vi "字符检测CCD1-1.vi"(8 "error in (no error)":errorcluster caption="错误输入（无错误）", 11 "名称或相对路径":string="Template Program") -> (0 "error in (no error) 2":errorcluster caption="错误输入（无错误）")   [LabVIEW 2017]
uses:
  Picture/SaveButtom.ctl
  Global System.vi
  <vilib>/Utility/xml.llb/Write to XML File(string).vi
panel:
  in  "获取图像":bool
  in  "ROI获取":bool
  in  "创建模板":bool
  in  "保存图像":bool
  out "添加的路径":path
  in  "刷新":bool
  in  "测试按钮":bool
  in  "保存按钮":bool
  in  "Main":enum32{"主参数", "字符检测参数 ", "测试效果"}(tab)
  in  "字符检测基础参数":T1={"IsNorImage"=TRUE, "Exposure Values"=100289, "ImagePath"=path "C:/Users/hedongpo/Desktop/514-hdp/Alignment Assemble System/Test Picture/B/3.bmp"} caption="参数界面" {"Exposure Values" scale=0.0..200000.0}
  in  "Angle (degrees)":sgl=93.5
  in  "字符识别参数":T3={"Parameters (OCR/OCV 1)"={"Threshold Data"={"Method"=enum."Local", "Looking for"=1, "Color Mode"=0, "Kernel Size"={"Width"=32, "Height"=32}, "Ranges"=[{"Min"=1, "Max"=255}]}, "Reject Border"=TRUE, "Number \nOf Erosions"=0, "Size & Spacing"={"Segment Algorithm"=0, "Min Bounding Rect Width"=1, "Max Bounding Rect Width"=65536, "Min Bounding Rect Height"=1, "Max Bounding Rect Height"=65536, "Min Character Size"=20, "Max Character Size"=65536, "Min Char Spacing"=1, "Max Horiz Element Spacing"=1, "Max Vert Element Spacing"=0, "Max Space Distance"=65536}, "Read Options"={"Read Strategy"=1, "Read Resolution"=2, "Scale Dependant"=FALSE, "Aspect Ratio"=400, "Acceptance Level"=700, "Substitution Character"="?", "MultiLine"=TRUE}, "Valid Characters"=[], "Use Text Pattern"=FALSE, "Orientation"=0, "# Lines Expected"=0, "Number of Blocks"=4}, "File Path "=path "D:/Inspect System -2/Source Code/Template Program/字符模板.abc", "Rectangle"={"Left"=0, "Top"=0, "Right"=0, "Bottom"=0, "Rotation"=0.0}, "字符长度判定"=0.0} {"Rectangle"."Rotation" min=-90.0 max=90.0 step=1.0 format="%.2f"; "Rectangle"."Left" scale=0.0..1024.0; "Rectangle"."Right" scale=0.0..1024.0; "Parameters (OCR/OCV 1)"."Threshold Data"."Looking for" items=["Light on Dark", "Dark on Light"]; "Parameters (OCR/OCV 1)"."Threshold Data"."Color Mode" items=["RGB", "HSL", "HSV", "HSI"]; "Parameters (OCR/OCV 1)"."Size & Spacing"."Segment Algorithm" items=["None", "Shortest Segment", "Legacy Auto Split"]; "Parameters (OCR/OCV 1)"."Read Options"."Read Strategy" items=["Aggressive", "Conservative"]; "Parameters (OCR/OCV 1)"."Read Options"."Read Resolution" items=["Low", "Medium", "High"]; "Parameters (OCR/OCV 1)"."Valid Characters"."Pre-defined characters" items=["Any Character", "User-defined Characters", "Alphabetic", "Alphanumeric", "Uppercase Letters", "Lowercase Letters", "Decimal Digits", "Hexadecimal Digits", "Pattern", "Force Space"]; "Parameters (OCR/OCV 1)"."Orientation" items=["Baseline inside", "Baseline outside"]}
  out "原始图像":T4(plugin-control)
  out "String (OCR/OCV 1)":string
  out "路径输出":path
  in  "Vision Paramter Save Buttom":T5
  out "system time":string
  in  "取消按钮":bool
  # "85"
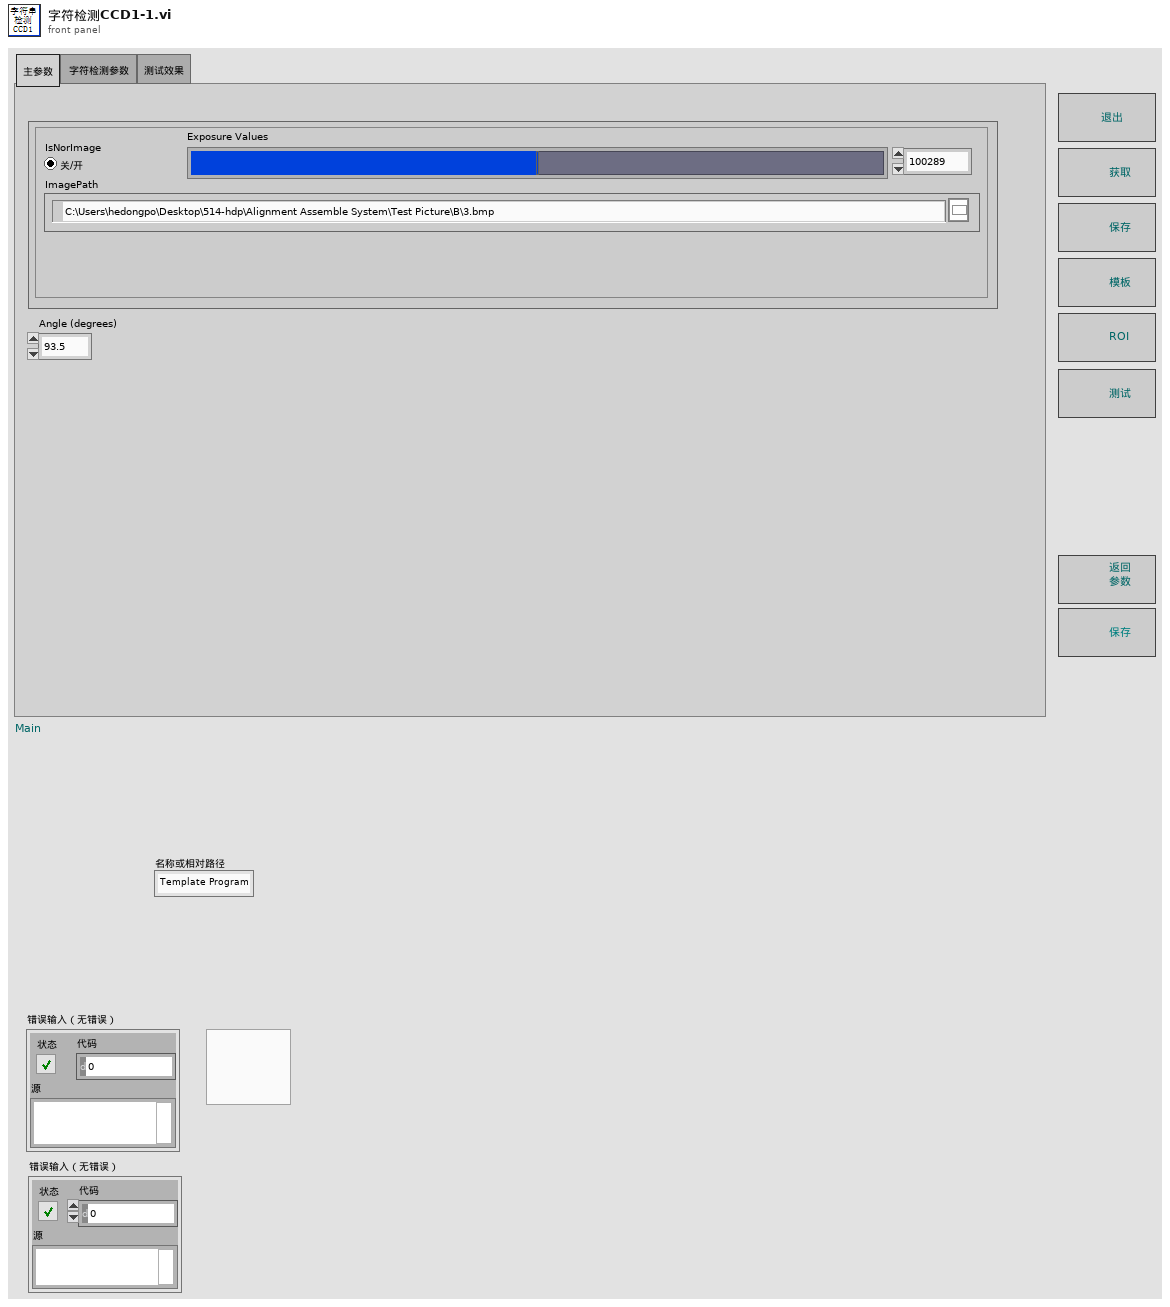
[diagram p1: front panel]
types:
  T1 = cluster{"IsNorImage":bool, "Exposure Values":u32, "ImagePath":path}
  T2 = typedef "IMAQ Rectangle" = cluster{"Left":i32, "Top":i32, "Right":i32, "Bottom":i32, "Rotation":dbl}
  T3 = cluster{"Parameters (OCR/OCV 1)":cluster{"Threshold Data":cluster{"Method":enum16{"Fixed Range", "Uniform", "Linear", "Non Linear", "Local", "Color"}, "Looking for":u32, "Color Mode":u32, "Kernel Size":cluster{"Width":i32, "Height":i32}, "Ranges":cluster{"Min":i32, "Max":i32}[]}, "Reject Border":bool, "Number \nOf Erosions":i32, "Size & Spacing":cluster{"Segment Algorithm":u16, "Min Bounding Rect Width":i32, "Max Bounding Rect Width":i32, "Min Bounding Rect Height":i32, "Max Bounding Rect Height":i32, "Min Character Size":i32, "Max Character Size":i32, "Min Char Spacing":i32, "Max Horiz Element Spacing":i32, "Max Vert Element Spacing":i32, "Max Space Distance":i32}, "Read Options":cluster{"Read Strategy":i32, "Read Resolution":i32, "Scale Dependant":bool, "Aspect Ratio":i32, "Acceptance Level":i32, "Substitution Character":string, "MultiLine":bool}, "Valid Characters":cluster{"Pre-defined characters":i32, "User-defined characters":string}[], "Use Text Pattern":bool, "Orientation":u32, "# Lines Expected":u32, "Number of Blocks":i32}, "File Path ":path, "Rectangle":T2, "字符长度判定":dbl}
  T4 = typedef "IMAQ Image.ctl" = refnum<image>
  T5 = typedef "SaveButtom.ctl" = bool
  T6 = cluster{"index":i32, "this vi":refnum<vi>, "error out":errorcluster}
  T7 = cluster{"master data":string, "priority":u16, "secondary data":string[]}
  T8 = cluster{"case name":string[], "queue array":refnum<queue>[]}
  T9 = cluster{"Global Rectangle":i32[], "Contours":cluster{"Contour Type":u32, "ROI Type":u32, "Points":i32[]}[]}
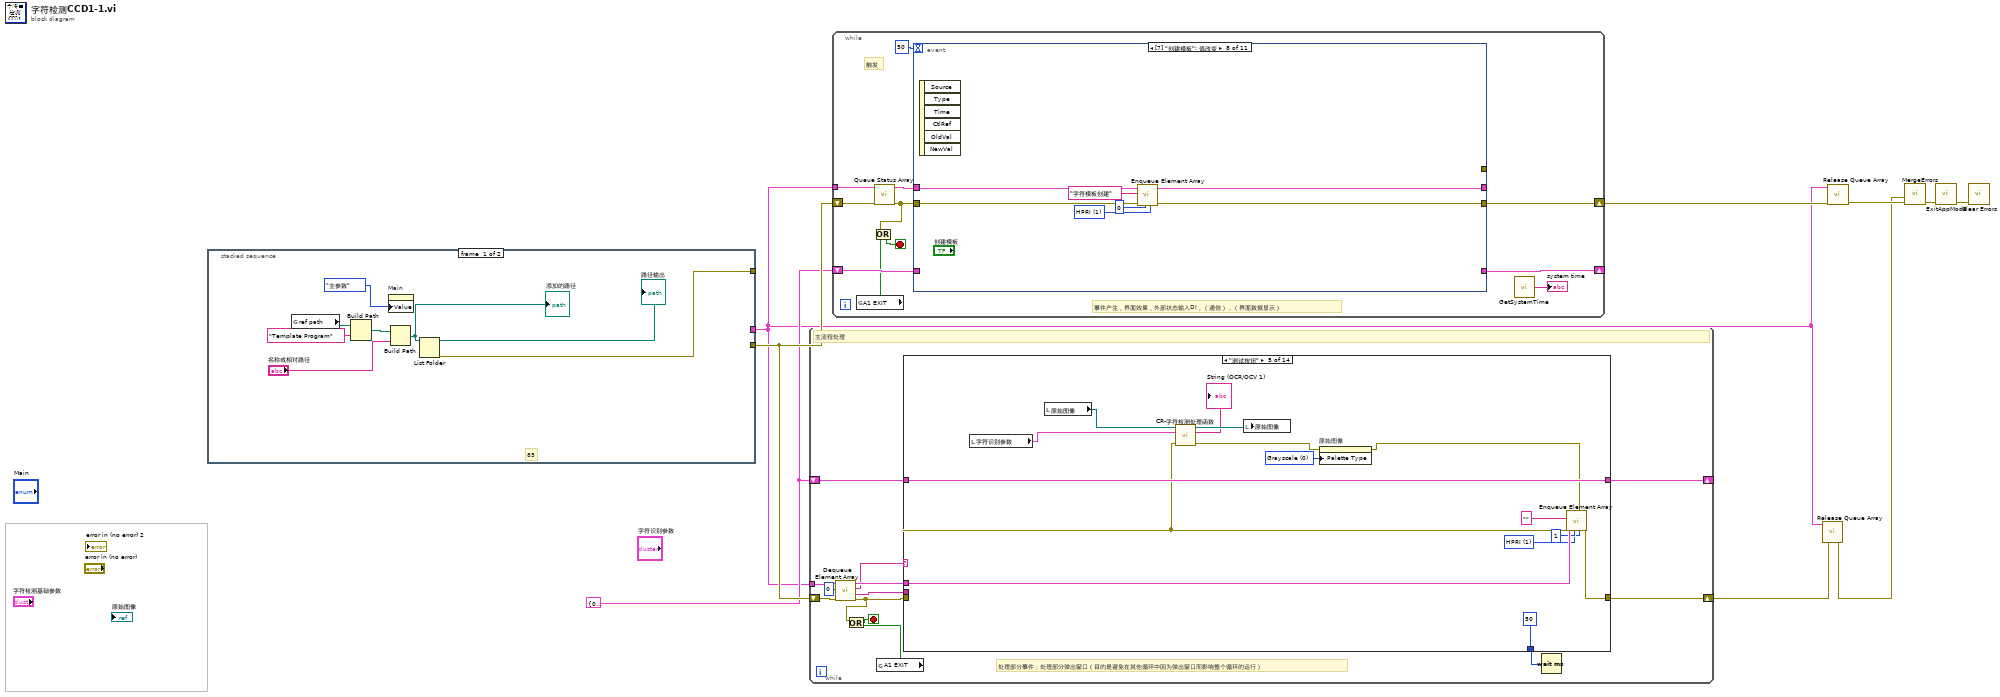
[diagram p0: block diagram]
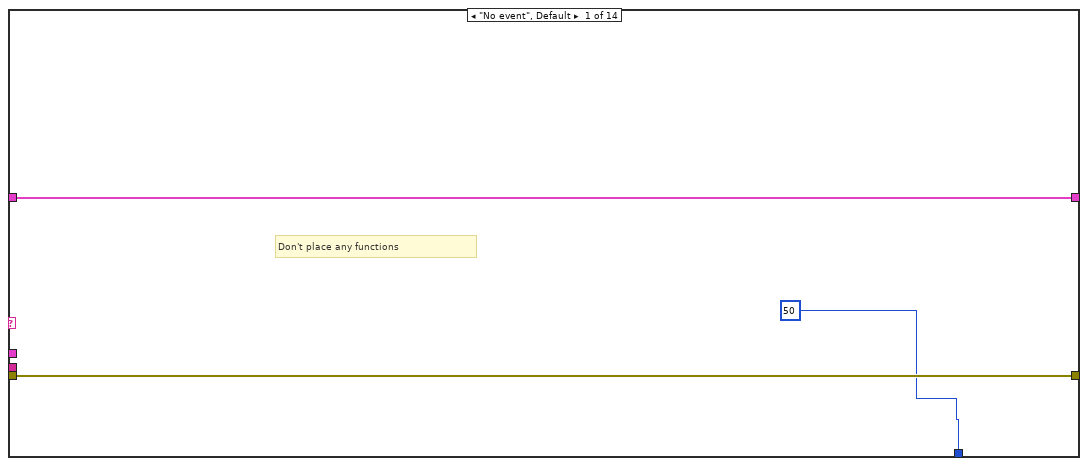
[diagram p2: hidden frame]
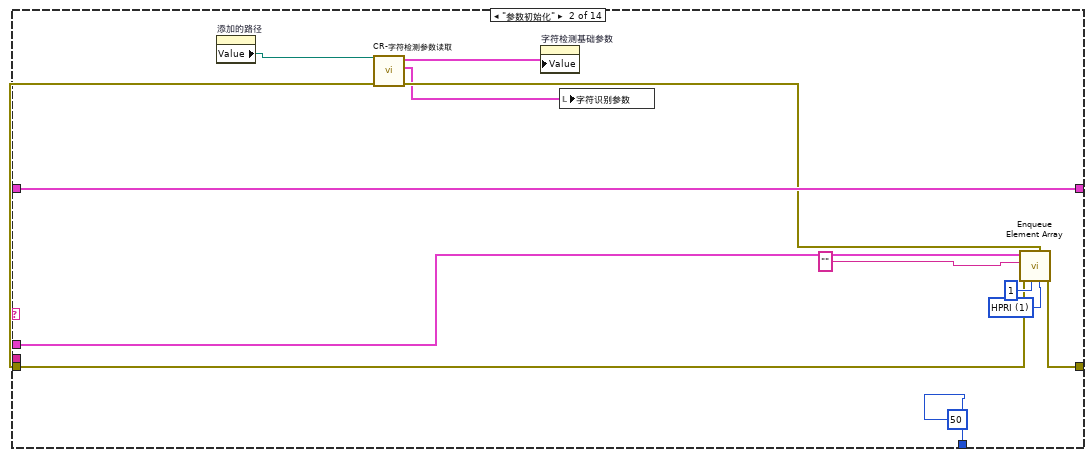
[diagram p3: hidden frame]
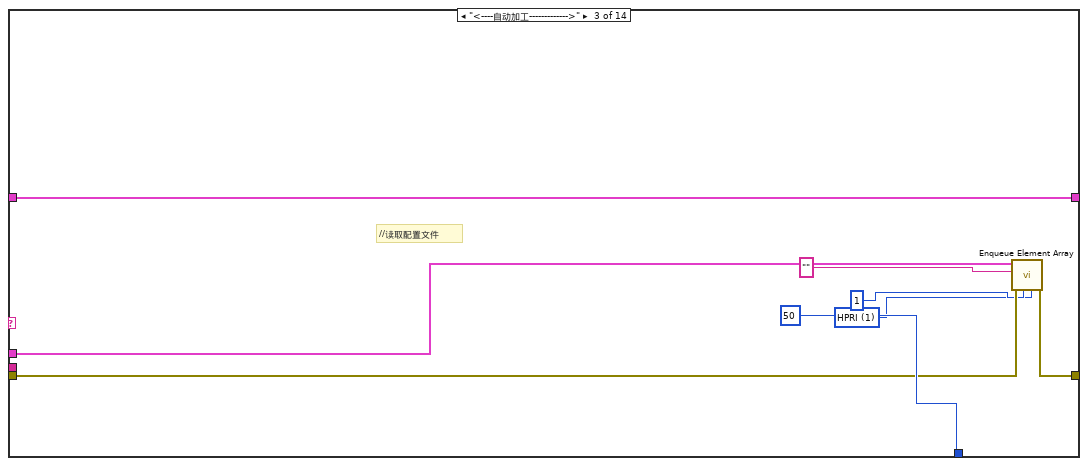
[diagram p4: hidden frame]
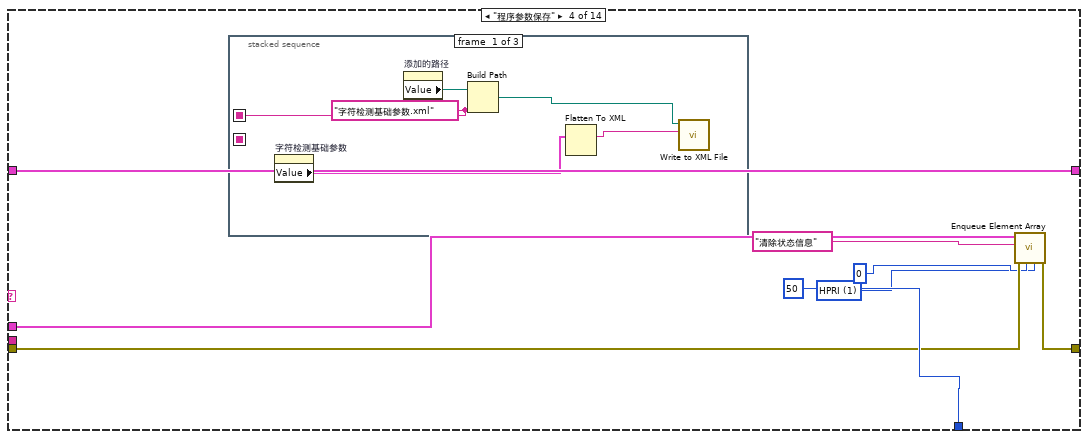
[diagram p5: hidden frame]
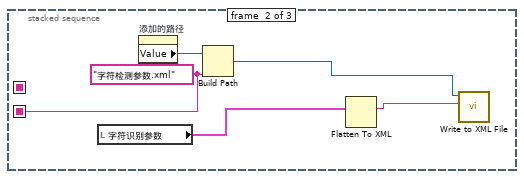
[diagram p6: hidden frame]
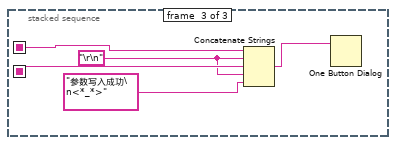
[diagram p7: hidden frame]
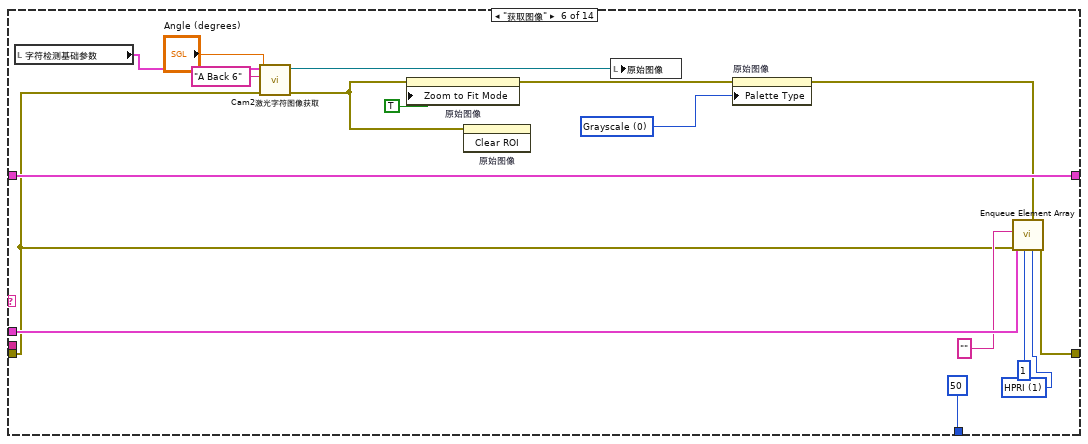
[diagram p8: hidden frame]
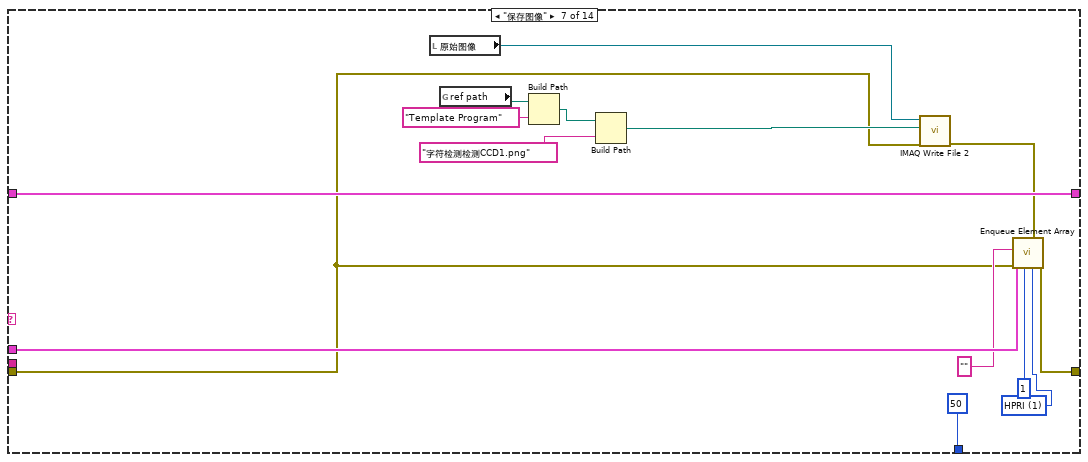
[diagram p9: hidden frame]
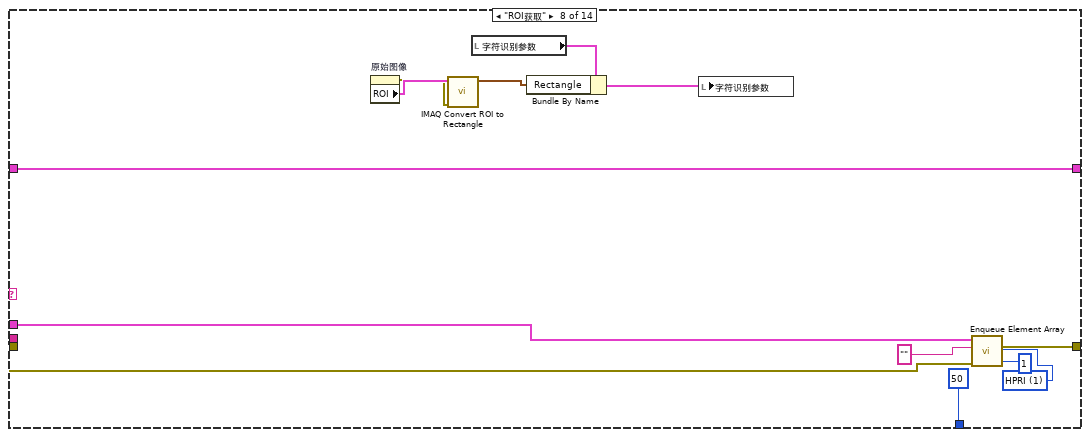
[diagram p10: hidden frame]
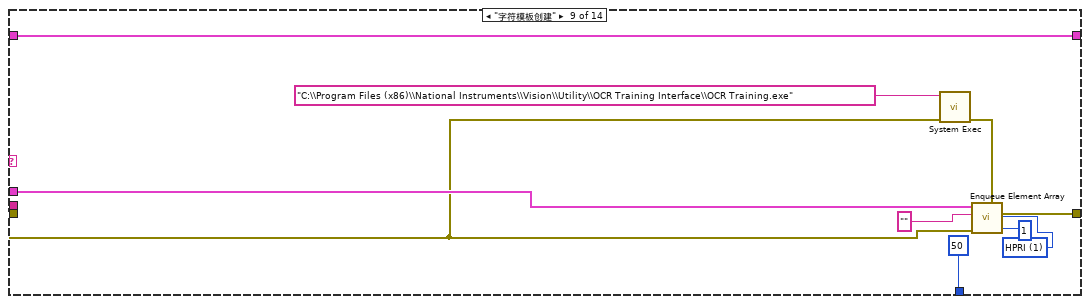
[diagram p11: hidden frame]
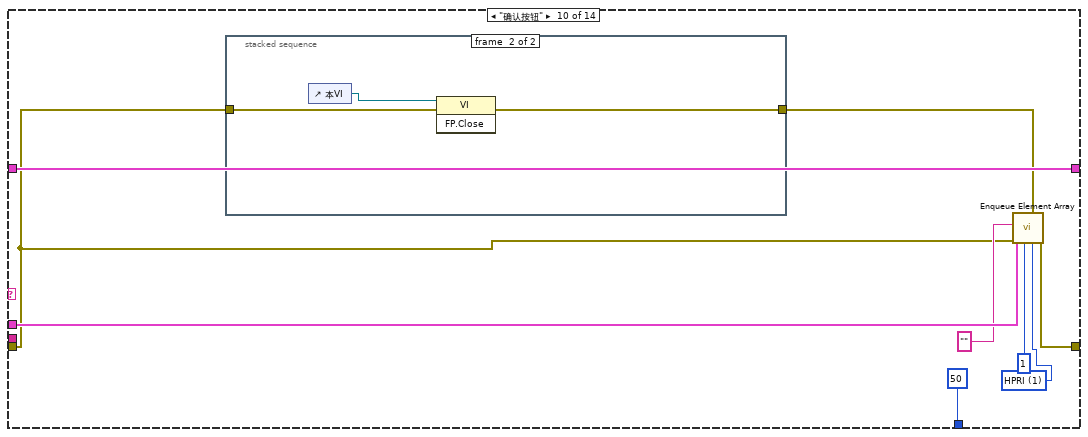
[diagram p12: hidden frame]
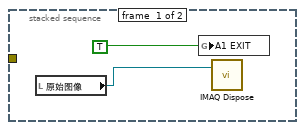
[diagram p13: hidden frame]
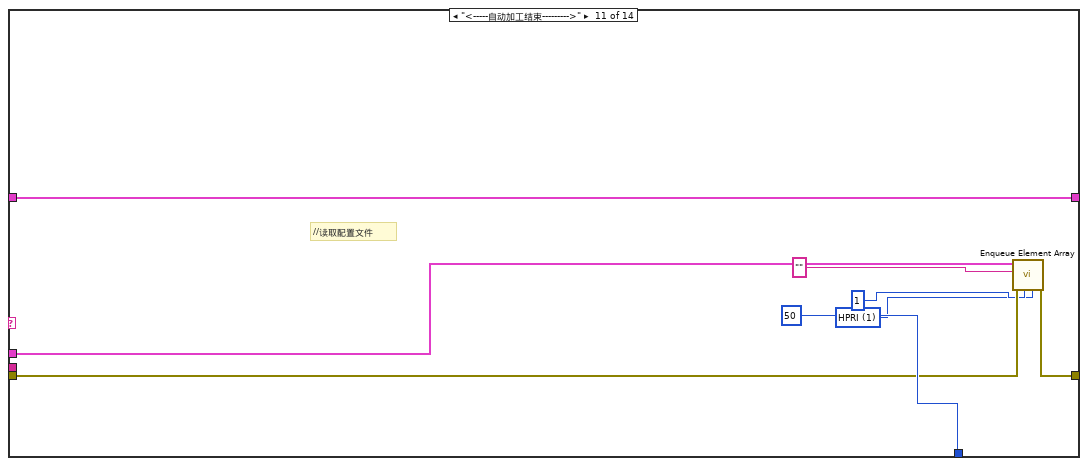
[diagram p14: hidden frame]
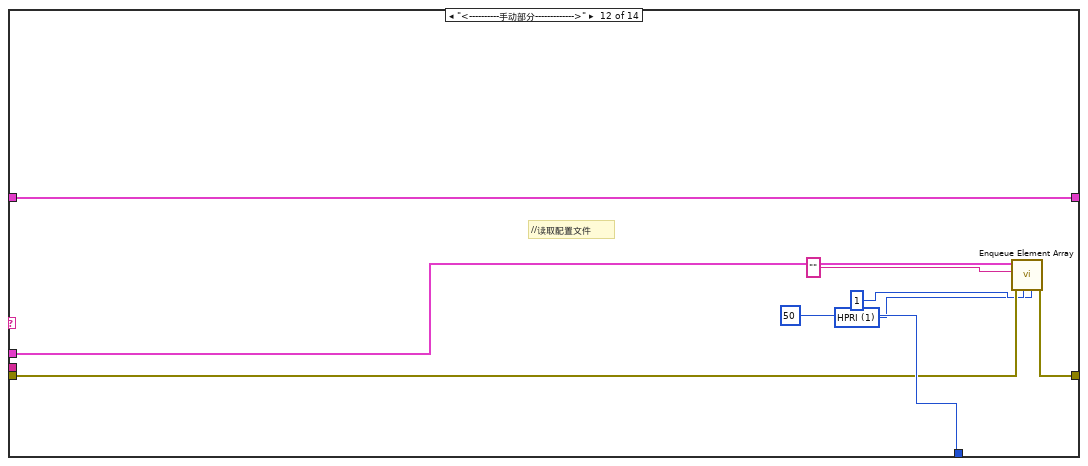
[diagram p15: hidden frame]
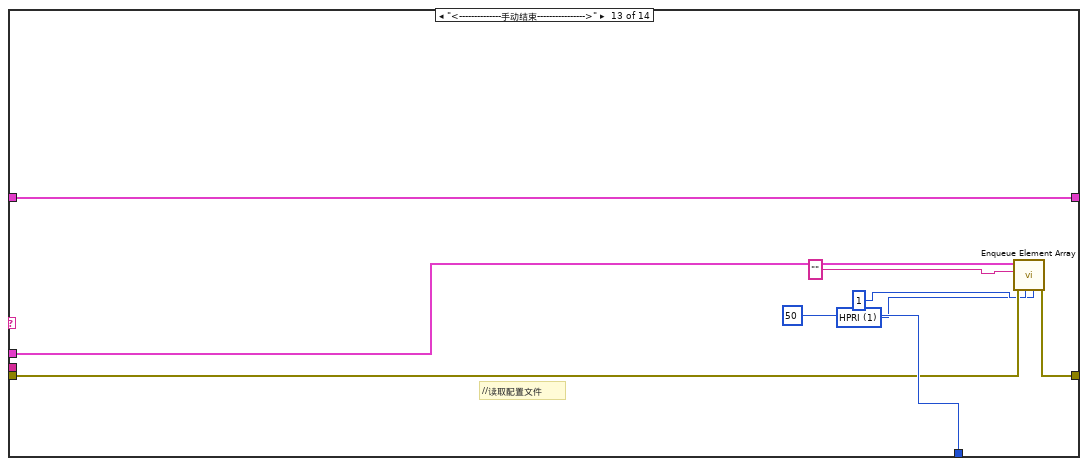
[diagram p16: hidden frame]
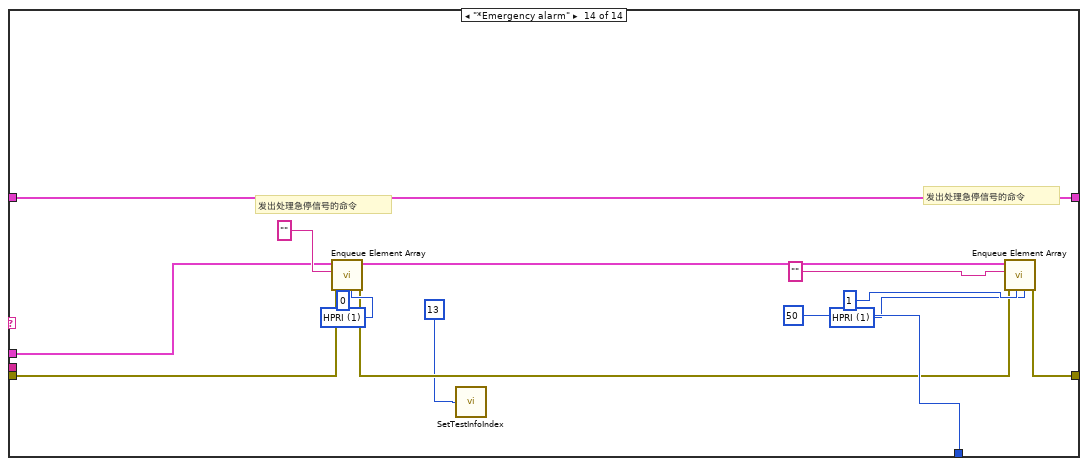
[diagram p17: hidden frame]
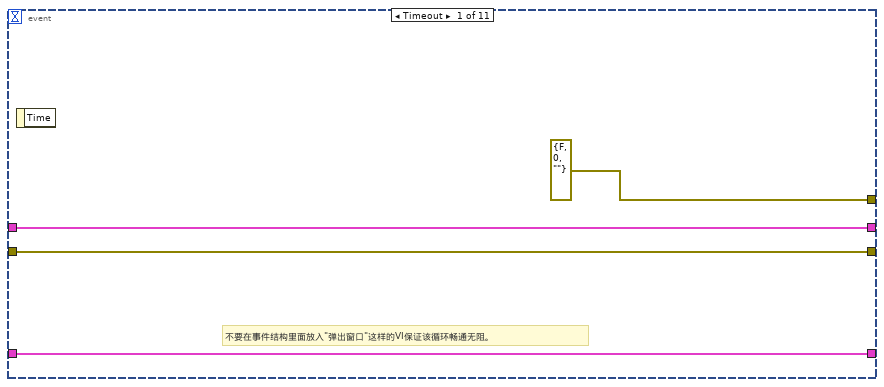
[diagram p18: hidden frame]
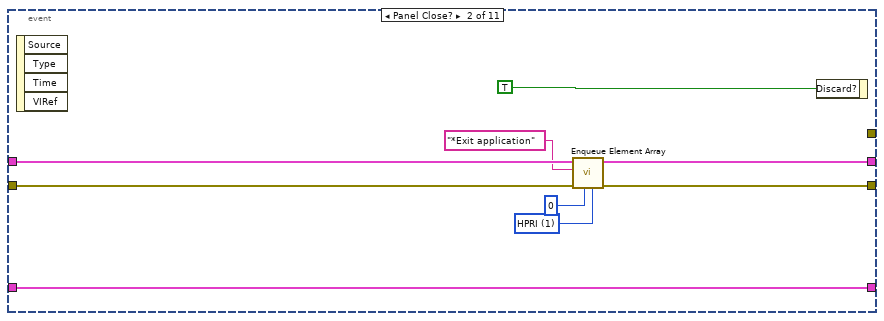
[diagram p19: hidden frame]
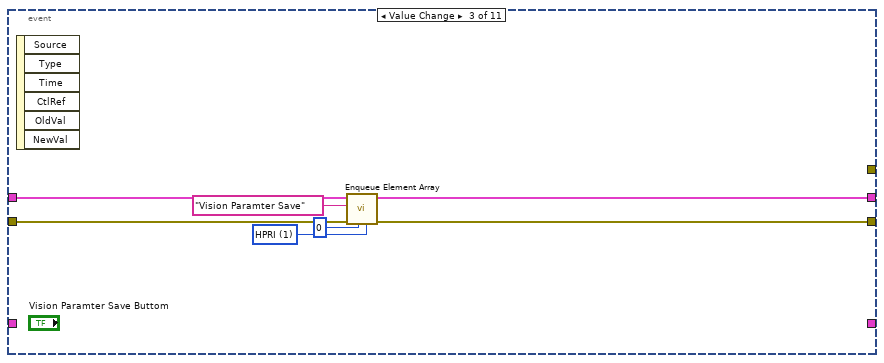
[diagram p20: hidden frame]
diagram:
  w4 = T6 {"index"=0, "this vi"=refnum, "error out"={"status"=FALSE, "code"=0, "source"=""}} ("parameter buffer")
  # "85"
  n1 = stacked-sequence {
    tunnel: [w15 _] -> _
    tunnel: [_ w19] -> w5
    tunnel: [_ w18] -> w1
    frame #0 {
      n2 = global read "Global System.vi" "ref path"() -> (w13:path)
      n3 = Build Path(base path=w13, name or relative path="Template Program" ("名称或相对路径")) -> (appended path=w11:path)
      n4 = property on="Main" class="TabCtl (严格)"("Value"=enum32{"主参数", "字符检测参数 ", "测试效果"}."主参数" ("Main")) -> ()  [unwired: 2 in, 2 out]
      n5 = Build Path(base path=w11, name or relative path="名称或相对路径") -> (appended path=w17:path)
      "添加的路径" <- w17
      n6 = List Folder(path=w17) -> (path out=→"路径输出":path, error out=w15:errorcluster)  [unwired: 3 in, 2 out]
    }
    frame #1 {
      w27 = string[] ["comm queue1", "data queue 11", "data queue 12", "data queue 13", "data queue 14"]  # queue name
      w28 = 4  # queue num
      w29 = T7 {"master data"="", "priority"=0, "secondary data"=[]}  # element data type
      n7 = call "Obtain Queue Array.vi"("queue name"=w27, "element data type"=w29, "queue num"=w28) -> ("error out"=w23:errorcluster, "queue out"=w24:T8)  [unwired: 2 in, 1 out]
      n8 = call "Enqueue Element Array.vi"("queue index"=0, "error in"=w23, "master data"="参数初始化", "queue in"=w24) -> ("error out"=w22:errorcluster, "queue out"=w21:T8)  [unwired: 6 in]
      n9 = disable-structure shown="启用" {
        disable-tunnel: w22 -> [w35 w36]
        disable-tunnel: w21 -> [w34 w37]
        disable-tunnel: "Loading Variable" ("master data") -> [w33 _]
        disable-tunnel: [w31 w36] -> w19
        disable-tunnel: [w30 w37] -> w18
        frame Disabled {
          n10 = call "Enqueue Element Array.vi"("queue index"=12, "error in"=w35, "master data"=w33, "queue in"=w34) -> ("error out"=w31:errorcluster, "queue out"=w30:T8)  [unwired: 6 in]
        }
        frame Enabled {
        }
      }
    }
  }
  n11 = while {
    shift-right: [w50] -> w3
    shift-left: w5 -> [w41]
    shift-right: [w47] -> _
    shift-left: w4 -> [w48]
    tunnel: w1 -> [w43]
    stop <- w38 stop-if-true
    # "处理部分事件；处理部分弹出窗口（目的是避免在其他循环中因为弹出窗口而影响整个循环的运行）"
    # "主流程处理"
    n12 = call "Dequeue Element Array.vi"("queue in"=w43, "queue index"=0, "error in"=w41) -> ("queue out"=w46:T8, "master data"=w45:string, "secondary data"=w44:string[], "error out"=w40:errorcluster)  [unwired: 2 in, 1 out]
    n13 = global read "Global System.vi" "A1 EXIT"() -> (w39:bool)
    n14 = Or(x=w40, y=w39) -> (x .or. y?=w38:bool)
    n15 = case shown="\"测试按钮\"" w45 {
      tunnel: w46 -> [_ w64 w72 w74 w110 w127 w142 w155 w165 w174 w187 w195 w203 w209]
      tunnel: w40 -> [w52 w58 w68 w78 w104 w118 w130 w149 w159 w168 w183 w191 w199 w206]
      tunnel: [w52 w63 w71 w80 w109 w126 w141 w154 w164 w173 w186 w194 w202 w217] -> w50
      tunnel: [50 50 50 50 50 50 50 50 50 50 50 50 50 50] -> w49
      tunnel: w48 -> [w53 w59 w69 w75 w105 w122 w137 w150 w160 w169 w184 w192 w200 w215]
      tunnel: [w53 w59 w69 w75 w105 w122 w137 w150 w160 w169 w184 w192 w200 w215] -> w47
      tunnel: w44 -> [_ _ _ _ _ _ _ _ _ _ _ _ _ _]
      frame "No event", Default {
        # "Don't place any functions"
      }
      frame "参数初始化" {
        w60 = u16 1 items=["HPRI"=1, "LPRI"=0] ("priority")
        n16 = property on="添加的路径" class="Path"() -> ("Value"=w56:path)  [unwired: 2 in, 2 out]
        n17 = call "CR-字符检测参数读取.vi"("error in (no error)"=w58, "基路径"=w56) -> ("error out"=w57:errorcluster, "字符识别参数"=w54:T3, "字符检测基础参数"=w55:T1)  [unwired: 6 in]
        n18 = property on="字符检测基础参数" class="Clust (严格)"("Value"=w55) -> ()  [unwired: 2 in, 2 out]
        n19 = local write "字符识别参数"(w54) -> ()
        n20 = call "Enqueue Element Array.vi"("priority"=w60, "device error in"=w57, "queue index"=1, "error in"=w58, "master data"="" ("Element 1"), "queue in"=w64) -> ("error out"=w63:errorcluster)  [unwired: 4 in, 1 out]
      }
      frame "<----自动加工------------->" {
        w66 = u16 1 items=["HPRI"=1, "LPRI"=0] ("priority")
        # "//读取配置文件"
        n21 = call "Enqueue Element Array.vi"("priority"=w66, "queue index"=1, "error in"=w68, "master data"="" ("Element 1"), "queue in"=w72) -> ("error out"=w71:errorcluster)  [unwired: 5 in, 1 out]
      }
      frame "程序参数保存" {
        w76 = u16 1 items=["HPRI"=1, "LPRI"=0] ("priority")
        n22 = stacked-sequence {
          seq-local: [w82 _ _] -> [_ _ w95]
          seq-local: [_ w91 _] -> [_ _ w93]
          frame #0 {
            w82 = "字符检测基础参数.xml" ("名称或相对路径")
            n23 = property on="字符检测基础参数" class="Clust (严格)"() -> ("Value"=w85:T1)  [unwired: 2 in, 2 out]
            n24 = property on="添加的路径" class="Path"() -> ("Value"=w86:path)  [unwired: 2 in, 2 out]
            n25 = Build Path(base path=w86, name or relative path=w82) -> (appended path=w83:path)
            n26 = Flatten To XML(anything=w85) -> (xml string=w84:string)
            n27 = call-poly <vilib>:"Write to XML File.vi"("XML Input"=w84, "XML File Path"=w83) -> ()  [unwired: 7 in, 3 out]
          }
          frame #1 {
            w91 = "字符检测参数.xml" ("名称或相对路径")
            n28 = local read "字符识别参数"() -> (w87:T3)
            n29 = property on="添加的路径" class="Path"() -> ("Value"=w90:path)  [unwired: 2 in, 2 out]
            n30 = Build Path(base path=w90, name or relative path=w91) -> (appended path=w88:path)
            n31 = Flatten To XML(anything=w87) -> (xml string=w89:string)
            n32 = call-poly <vilib>:"Write to XML File.vi"("XML Input"=w89, "XML File Path"=w88) -> ()  [unwired: 7 in, 3 out]
          }
          frame #2 {
            w92 = "\r\n"
            n33 = Concatenate Strings(w95, w92, w93, w92, "参数写入成功\n<*_*>" ("消息")) -> (w94:string)
            n34 = One Button Dialog(message=w94) -> ()  [unwired: 1 in, 1 out]
          }
        }
        n35 = call "Enqueue Element Array.vi"("priority"=w76, "queue index"=0, "error in"=w78, "master data"="清除状态信息" ("Element 1"), "queue in"=w74) -> ("error out"=w80:errorcluster)  [unwired: 5 in, 1 out]
      }
      frame "测试按钮" {
        w100 = u32 0 items=["Grayscale", "Binary", "Gradient", "Rainbow", "Temperature", "User Defined", "Binary 16 Bit", "Gradient 16 Bit", "Rainbow 16 Bit", "Temperature 16 Bit", "User Defined 16 Bit"] ("Palette:Palette Type")
        w106 = u16 1 items=["HPRI"=1, "LPRI"=0] ("priority")
        n36 = local read "字符识别参数"() -> (w97:T3)
        n37 = local read "原始图像"() -> (w101:T4)
        n38 = call "CR-字符检测处理函数.vi"("error in (no error)"=w104, "字符识别参数"=w97, "Image in"=w101) -> ("error out"=w99:errorcluster, "String (OCR/OCV 1)"=→"String (OCR/OCV 1)":string, "Image out"=w103:T4)  [unwired: 4 in, 2 out]
        n39 = local write "原始图像"(w103) -> ()
        n40 = property on="原始图像" class="ImageControl"(error in=w99, "Palette Type"=w100) -> (error out=w98:errorcluster)  [unwired: 1 in, 1 out]
        n41 = call "Enqueue Element Array.vi"("priority"=w106, "device error in"=w98, "queue index"=1, "error in"=w104, "master data"="" ("Element 1"), "queue in"=w110) -> ("error out"=w109:errorcluster)  [unwired: 4 in, 1 out]
      }
      frame "获取图像" {
        w115 = u32 0 items=["Grayscale", "Binary", "Gradient", "Rainbow", "Temperature", "User Defined", "Binary 16 Bit", "Gradient 16 Bit", "Rainbow 16 Bit", "Temperature 16 Bit", "User Defined 16 Bit"] ("Palette:Palette Type")
        w123 = u16 1 items=["HPRI"=1, "LPRI"=0] ("priority")
        n42 = local read "字符检测基础参数"() -> (w120:T1)
        n43 = call "Cam2激光字符图像获取.vi"("error in (no error)"=w118, "Angle (degrees)"="Angle (degrees)", "Image Name"="A Back 6", "ParamsUI"=w120) -> ("error out"=w116:errorcluster, "Image out"=w119:T4)  [unwired: 3 in, 3 out]
        n44 = property on="原始图像" class="ImageControl"(error in=w116, "Zoom to Fit Mode"=TRUE) -> (error out=w114:errorcluster)  [unwired: 1 in, 1 out]
        n45 = invoke on="原始图像" class="ImageControl" method="Clear ROI"(error in=w116) -> ()  [unwired: 2 in, 3 out]
        n46 = local write "原始图像"(w119) -> ()
        n47 = property on="原始图像" class="ImageControl"(error in=w114, "Palette Type"=w115) -> (error out=w113:errorcluster)  [unwired: 1 in, 1 out]
        n48 = call "Enqueue Element Array.vi"("priority"=w123, "device error in"=w113, "queue index"=1, "error in"=w118, "master data"="" ("Element 1"), "queue in"=w127) -> ("error out"=w126:errorcluster)  [unwired: 4 in, 1 out]
      }
      frame "保存图像" {
        w138 = u16 1 items=["HPRI"=1, "LPRI"=0] ("priority")
        n49 = local read "原始图像"() -> (w129:T4)
        n50 = global read "Global System.vi" "ref path"() -> (w136:path)
        n51 = Build Path(base path=w136, name or relative path="Template Program" ("名称或相对路径")) -> (appended path=w134:path)
        n52 = Build Path(base path=w134, name or relative path="字符检测检测CCD1.png" ("名称或相对路径")) -> (appended path=w132:path)
        n53 = call-poly "IMAQ Write File 2"("error in (no error)"=w130, "File Path"=w132, "Image"=w129) -> ("error out"=w131:errorcluster)  [unwired: 7 in, 1 out]
        n54 = call "Enqueue Element Array.vi"("priority"=w138, "device error in"=w131, "queue index"=1, "error in"=w130, "master data"="" ("Element 1"), "queue in"=w142) -> ("error out"=w141:errorcluster)  [unwired: 4 in, 1 out]
      }
      frame "ROI获取" {
        w151 = u16 1 items=["HPRI"=1, "LPRI"=0] ("priority")
        n55 = property on="原始图像" class="ImageControl"() -> (error out=w145:errorcluster, "ROI"=w146:T9)  [unwired: 2 in, 1 out]
        n56 = call "IMAQ Convert ROI to Rectangle"("error in (no error)"=w145, "ROI Descriptor"=w146) -> ("Rectangle"=w144:T2)  [unwired: 7 in, 1 out]
        n57 = local read "字符识别参数"() -> (w148:T3)
        n58 = Bundle By Name(cluster=w148, "Rectangle"=w144) -> (w147:T3)
        n59 = local write "字符识别参数"(w147) -> ()
        n60 = call "Enqueue Element Array.vi"("priority"=w151, "queue index"=1, "error in"=w149, "master data"="" ("Element 1"), "queue in"=w155) -> ("error out"=w154:errorcluster)  [unwired: 5 in, 1 out]
      }
      frame "字符模板创建" {
        w161 = u16 1 items=["HPRI"=1, "LPRI"=0] ("priority")
        n61 = call <vilib>:"System Exec.vi"("error in (no error)"=w159, "command line"="C:\\Program Files (x86)\\National Instruments\\Vision\\Utility\\OCR Training Interface\\OCR Training.exe") -> ("error out"=w158:errorcluster)  [unwired: 6 in, 3 out]
        n62 = call "Enqueue Element Array.vi"("priority"=w161, "device error in"=w158, "queue index"=1, "error in"=w159, "master data"="" ("Element 1"), "queue in"=w165) -> ("error out"=w164:errorcluster)  [unwired: 4 in, 1 out]
      }
      frame "确认按钮" {
        w170 = u16 1 items=["HPRI"=1, "LPRI"=0] ("priority")
        n63 = stacked-sequence {
          tunnel: w168 -> [_ w179]
          tunnel: [_ w178] -> w167
          frame #0 {
            n64 = local read "原始图像"() -> (w176:T4)
            n65 = global write "Global System.vi" "A1 EXIT"(TRUE ("EXIT")) -> ()
            n66 = call "IMAQ Dispose"("Image"=w176) -> ()  [unwired: 5 in, 1 out]
          }
          frame #1 {
            n67 = control-ref of="本VI"() -> (w180:refnum<vi>)
            n68 = invoke class="VI" method="FP.Close"(reference=w180, error in=w179) -> (error out=w178:errorcluster)  [unwired: 1 in, 2 out]
          }
        }
        n69 = call "Enqueue Element Array.vi"("priority"=w170, "device error in"=w167, "queue index"=1, "error in"=w168, "master data"="" ("Element 1"), "queue in"=w174) -> ("error out"=w173:errorcluster)  [unwired: 4 in, 1 out]
      }
      frame "<-----自动加工结束--------->" {
        w181 = u16 1 items=["HPRI"=1, "LPRI"=0] ("priority")
        # "//读取配置文件"
        n70 = call "Enqueue Element Array.vi"("priority"=w181, "queue index"=1, "error in"=w183, "master data"="" ("Element 1"), "queue in"=w187) -> ("error out"=w186:errorcluster)  [unwired: 5 in, 1 out]
      }
      frame "<----------手动部分------------->" {
        w189 = u16 1 items=["HPRI"=1, "LPRI"=0] ("priority")
        # "//读取配置文件"
        n71 = call "Enqueue Element Array.vi"("priority"=w189, "queue index"=1, "error in"=w191, "master data"="" ("Element 1"), "queue in"=w195) -> ("error out"=w194:errorcluster)  [unwired: 5 in, 1 out]
      }
      frame "<--------------手动结束---------------->" {
        w197 = u16 1 items=["HPRI"=1, "LPRI"=0] ("priority")
        # "//读取配置文件"
        n72 = call "Enqueue Element Array.vi"("priority"=w197, "queue index"=1, "error in"=w199, "master data"="" ("Element 1"), "queue in"=w203) -> ("error out"=w202:errorcluster)  [unwired: 5 in, 1 out]
      }
      frame "*Emergency alarm" {
        w212 = u16 1 items=["HPRI"=1, "LPRI"=0] ("priority")
        w213 = u16 1 items=["HPRI"=1, "LPRI"=0] ("priority")
        # "发出处理急停信号的命令"
        # "发出处理急停信号的命令"
        n73 = call "Enqueue Element Array.vi"("priority"=w212, "queue index"=0, "error in"=w206, "master data"="" ("Element 1"), "queue in"=w209) -> ("error out"=w207:errorcluster, "queue out"=w208:T8)  [unwired: 5 in]
        n74 = call "SetTestInfoIndex.vi"("test info index"=13) -> ()
        n75 = call "Enqueue Element Array.vi"("priority"=w213, "queue index"=1, "error in"=w207, "master data"="" ("Element 1"), "queue in"=w208) -> ("error out"=w217:errorcluster)  [unwired: 5 in, 1 out]
      }
    }
    n76 = Wait (ms)(milliseconds to wait=w49) -> ()  [unwired: 1 out]
  }
  n77 = while {
    shift-right: [w222] -> w6
    shift-left: w5 -> [w226]
    shift-right: [w224] -> _
    shift-left: w4 -> [w225]
    tunnel: w1 -> [w228]
    stop <- w219 stop-if-true
    # "触发"
    # "事件产生，界面效果，外部状态输入DI，（通信），（界面数据显示）"
    n78 = global read "Global System.vi" "A1 EXIT"() -> (w220:bool)
    n79 = call "Queue Status Array.vi"("error in (no error)"=w226, "queue in"=w228) -> ("error out"=w221:errorcluster, "queue out"=w223:T8)  [unwired: 4 in]
    n80 = Or(x=w221, y=w220) -> (x .or. y?=w219:bool)
    n81 = event shown="[7] \"创建模板\": 值改变" {
      selector: _ -> [_ _ _ _ _ _ _ _ _ _ _]
      dyn-events: _ -> [_ _ _ _ _ _ _ _ _ _ _]
      timeout: 50 -> [_ _ _ _ _ _ _ _ _ _ _]
      tunnel: w225 -> [w233 w241 _ _ _ _ _ _ _ _ _]
      tunnel: [w233 w241 _ _ _ _ _ _ _ _ _] -> w224
      tunnel: [errorcluster {"status"=FALSE, "code"=0, "source"=""} ("error out") _ _ _ _ _ _ _ _ _ _] -> _
      tunnel: w223 -> [w231 w240 w246 w253 w260 w268 w275 w282 w290 w298 w306]
      tunnel: w221 -> [w230 w239 w245 w252 w259 w267 w274 w281 w289 w297 w305]
      tunnel: [w230 w238 w243 w250 w257 w265 w272 w279 w287 w295 w303] -> w222
      tunnel: [w231 w237 w244 w251 w258 w266 w273 w280 w288 w296 w304] -> _
      event Timeout {
        # "不要在事件结构里面放入\"弹出窗口\"这样的VI保证该循环畅通无阻。"
        n82 = event-data() -> ()  [unwired: 1 in, 1 out]
      }
      event Panel Close? {
        w235 = u16 1 items=["HPRI"=1, "LPRI"=0] ("priority")
        n83 = event-data() -> ()  [unwired: 1 in, 4 out]
        n84 = call "Enqueue Element Array.vi"("priority"=w235, "queue index"=0, "error in"=w239, "master data"="*Exit application", "queue in"=w240) -> ("error out"=w238:errorcluster, "queue out"=w237:T8)  [unwired: 5 in]
        n85 = event-data("Discard?"=TRUE) -> ()  [unwired: 1 in, 1 out]
      }
      event Value Change {
        w248 = u16 1 items=["HPRI"=1, "LPRI"=0] ("priority")
        n86 = event-data() -> ()  [unwired: 1 in, 6 out]
        n87 = call "Enqueue Element Array.vi"("priority"=w248, "queue index"=0, "error in"=w245, "master data"="Vision Paramter Save", "queue in"=w246) -> ("error out"=w243:errorcluster, "queue out"=w244:T8)  [unwired: 5 in]
      }
      event "取消按钮": Value Change {
        w255 = u16 1 items=["HPRI"=1, "LPRI"=0] ("priority")
        n88 = event-data() -> ()  [unwired: 1 in, 6 out]
        n89 = call "Enqueue Element Array.vi"("priority"=w255, "queue index"=0, "error in"=w252, "master data"="确认按钮", "queue in"=w253) -> ("error out"=w250:errorcluster, "queue out"=w251:T8)  [unwired: 5 in]
      }
      event "保存按钮": Value Change {
        w262 = u16 1 items=["HPRI"=1, "LPRI"=0] ("priority")
        n90 = event-data() -> ()  [unwired: 1 in, 6 out]
        n91 = call "Enqueue Element Array.vi"("priority"=w262, "queue index"=0, "error in"=w259, "master data"="程序参数保存", "queue in"=w260) -> ("error out"=w257:errorcluster, "queue out"=w258:T8)  [unwired: 5 in]
      }
      event "获取图像": Value Change {
        w270 = u16 1 items=["HPRI"=1, "LPRI"=0] ("priority")
        n92 = event-data() -> ()  [unwired: 1 in, 6 out]
        n93 = property on="Main" class="TabCtl (严格)"("Value"=enum32{"主参数", "字符检测参数 ", "测试效果"}."测试效果" ("Main")) -> ()  [unwired: 2 in, 2 out]
        n94 = call "Enqueue Element Array.vi"("priority"=w270, "queue index"=0, "error in"=w267, "master data"="获取图像", "queue in"=w268) -> ("error out"=w265:errorcluster, "queue out"=w266:T8)  [unwired: 5 in]
      }
      event "保存图像": Value Change {
        w277 = u16 1 items=["HPRI"=1, "LPRI"=0] ("priority")
        n95 = event-data() -> ()  [unwired: 1 in, 6 out]
        n96 = call "Enqueue Element Array.vi"("priority"=w277, "queue index"=0, "error in"=w274, "master data"="保存图像", "queue in"=w275) -> ("error out"=w272:errorcluster, "queue out"=w273:T8)  [unwired: 5 in]
      }
      event "创建模板": Value Change {
        w284 = u16 1 items=["HPRI"=1, "LPRI"=0] ("priority")
        n97 = event-data() -> ()  [unwired: 1 in, 6 out]
        n98 = call "Enqueue Element Array.vi"("priority"=w284, "queue index"=0, "error in"=w281, "master data"="字符模板创建", "queue in"=w282) -> ("error out"=w279:errorcluster, "queue out"=w280:T8)  [unwired: 5 in]
      }
      event "ROI获取": Value Change {
        w292 = u16 1 items=["HPRI"=1, "LPRI"=0] ("priority")
        n99 = event-data() -> ()  [unwired: 1 in, 6 out]
        n100 = property on="Main" class="TabCtl (严格)"("Value"=enum32{"主参数", "字符检测参数 ", "测试效果"}."字符检测参数 " ("Main")) -> ()  [unwired: 2 in, 2 out]
        n101 = call "Enqueue Element Array.vi"("priority"=w292, "queue index"=0, "error in"=w289, "master data"="ROI获取", "queue in"=w290) -> ("error out"=w287:errorcluster, "queue out"=w288:T8)  [unwired: 5 in]
      }
      event "测试按钮": Value Change {
        w300 = u16 1 items=["HPRI"=1, "LPRI"=0] ("priority")
        n102 = event-data() -> ()  [unwired: 1 in, 6 out]
        n103 = property on="Main" class="TabCtl (严格)"("Value"=enum32{"主参数", "字符检测参数 ", "测试效果"}."测试效果" ("Main")) -> ()  [unwired: 2 in, 2 out]
        n104 = call "Enqueue Element Array.vi"("priority"=w300, "queue index"=0, "error in"=w297, "master data"="测试按钮", "queue in"=w298) -> ("error out"=w295:errorcluster, "queue out"=w296:T8)  [unwired: 5 in]
      }
      event "刷新": Value Change {
        n105 = event-data() -> ()  [unwired: 1 in, 6 out]
        n106 = disable-structure shown="禁用" {
          disable-tunnel: w306 -> [w310 _]
          disable-tunnel: w305 -> [w309 _]
          disable-tunnel: [w308 _] -> w304
          disable-tunnel: [w307 _] -> w303
          frame Disabled {
            w312 = u16 1 items=["HPRI"=1, "LPRI"=0] ("priority")
            # "刷新"
            n107 = call "Enqueue Element Array.vi"("priority"=w312, "queue index"=0, "error in"=w309, "master data"="刷新", "queue in"=w310) -> ("error out"=w307:errorcluster, "queue out"=w308:T8)  [unwired: 5 in]
          }
          frame Enabled {
          }
        }
        n108 = property on="Main" class="TabCtl (严格)"("Value"=enum32{"主参数", "字符检测参数 ", "测试效果"}."字符检测参数 " ("Main")) -> ()  [unwired: 2 in, 2 out]
      }
    }
    n109 = call "GetSystemTime.vi"() -> ("date/time string"=→"system time":string)  [unwired: 7 in]
  }
  n110 = call "Release Queue Array.vi"("error in"=w3, "queue in"=w1) -> ("error out"=w2:errorcluster)  [unwired: 2 in, 3 out]
  n111 = call "Release Queue Array.vi"("error in"=w6, "queue in"=w1) -> ("error out"=w9:errorcluster)  [unwired: 2 in, 3 out]
  n112 = call "MergeErrors.vi"("error in 3 (no error)"=w2, "error in 4 (no error)"=w9) -> ("error out"=w8:errorcluster)  [unwired: 6 in]
  n113 = call "ExitAppMode.vi"("error in (no error)"=w8) -> ("error out"=w7:errorcluster)  [unwired: 10 in]
  n114 = call <vilib>:"Clear Errors.vi"("error in (no error)"=w7) -> ()  [unwired: 5 in, 2 out]
